vi "macro_NumCmd_Recv_TwoDbl.vi"() -> ()   [LabVIEW 2019, in "Trajectory_Library.lvlib"]
uses:
  Trajectory_Library.lvlib
  VI/numCmd_ObtainQueue_TwoDbl.vi
panel:
  out "RightWheelDmd-Ft/Sec":dbl
  out "LeftWheelDmd-Ft/Sec":dbl
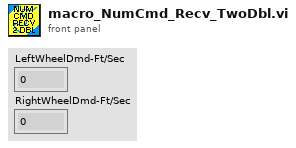
[diagram p1: front panel]
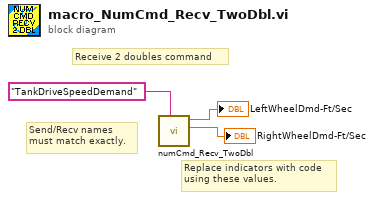
[diagram p0: block diagram]
diagram:
  # "Send/Recv names\nmust match exactly."
  # "Replace indicators with code\nusing these values."
  # "Receive 2 doubles command"
  n1 = call "numCmd_Recv_TwoDbl.vi"("Command Name"="TankDriveSpeedDemand") -> ("Value 2"=→"RightWheelDmd-Ft/Sec":dbl, "Value 1"=→"LeftWheelDmd-Ft/Sec":dbl)  [unwired: 7 in, 2 out]
